vi "SPD Stand Operator UI.vi"() -> ()   [LabVIEW 2018]
uses:
  Instruments/KC705 DevBoard/typedefs/DevB.Message type.ctl
  Instruments/KeySight 53230A/typedefs/FreqC.Message Type.ctl
  Instruments/KC705 DevBoard/Message API/Send Message/DevB.Send Message I32.vi
  Instruments/KC705 DevBoard/Message API/Get Data/Variant to I32.vi
  Instruments/KC705 DevBoard/Message API/Get Data/Variant to Bool.vi
  Instruments/SPD HID Interface/hidSPDLibForLabView/hidSPDLibForLabView.lvlib
panel:
  out "FCount.Connected":bool caption="Connected"
  out "SPD.HeatsinkTempChart":sgl(graph)=40.51374 caption="Heatsink Temprature"
  out "SPD.DiodTempChart":sgl(graph)=-42.149345 caption="Diod Temprature"
  out "FCount.Count":dbl caption="Count" format="%#_12p"
  in  "FCount.Timed Totalize":dbl caption="Totalize time" format="%#_g Sec"
  in  "FCount.Level":dbl caption="Threshold" format="%#_g V"
  out "DevB.Connected":bool caption="Connected"
  in  "DevB.Delay":i32 caption="Delay"
  in  "DevB.Phase":i32 caption="Phase"
  in  "DevB.Frequency":i32 caption="Frequency"
  in  "DevB.Pulse Duration":i32 caption="Duration"
  out "error out":errorcluster
  out "UI Stoped":bool
  in  "Stop":bool
  # "KC705 DevBoard"
  # "Counter"
  # "Photon Detector"
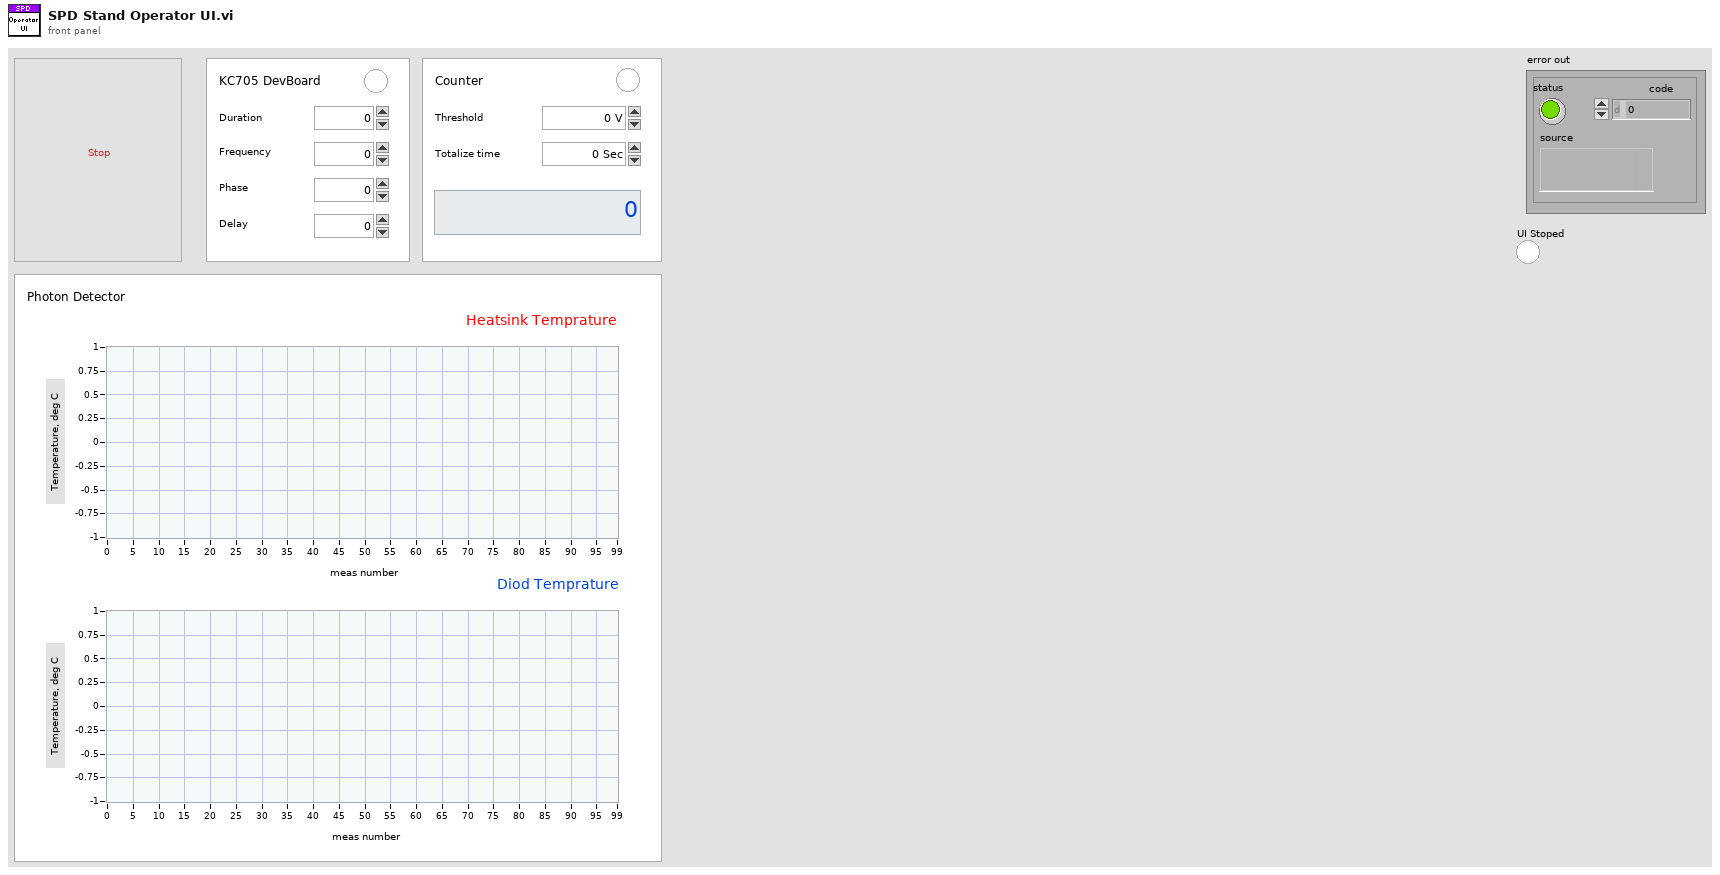
[diagram p1: front panel]
types:
  T1 = typedef "DevB.Message Session.ctl" = cluster{"Message queue":refnum<queue>, "stop event":refnum<user-event>}
  T2 = typedef "FreqC.Message Session.ctl" = cluster{"Message queue":refnum<queue>, "stop event":refnum<user-event>}
  T3 = typedef "hidSPDLibForLabView.lvlib/hidSPD HidDevInfo.ctl" = cluster{"name":string, "path":string}
  T4 = typedef "DevB.Session.ctl" = cluster{"DevBRef":refnum<visa-resource-name>, "connected":bool}
  T5 = typedef "hidSPDLibForLabView.lvlib/hidSPD Device Session.ctl" = cluster{"spdRef":u64, "connected":bool}
  T6 = typedef "FreqC.Session.ctl" = cluster{"FreqCRef":refnum<visa-resource-name>, "timeout":dbl, "connected":bool}
  T7 = typedef "DevB.Message type.ctl" = enum16{"Idle", "Set Duration", "Set Frequency", "Set Phase", "Set Delay", "on/off", "check status"}
  T8 = typedef "FreqC.Message Type.ctl" = enum16{"meas", "set level", "set gate"}
  T9 = typedef "hidSPDLibForLabView.lvlib/hidSPD Simple Report.ctl" = cluster{"Heatsink Temprature":sgl, "Diod Temprature":sgl, "TEC-voltage":sgl, "Diod Bias":sgl, "RF Power":sgl, "Thermal used":sgl, "hv bias used":sgl, "hv code used":u16, "strobe code used":u16, "SPD number":u8, "SPD ready":u8}
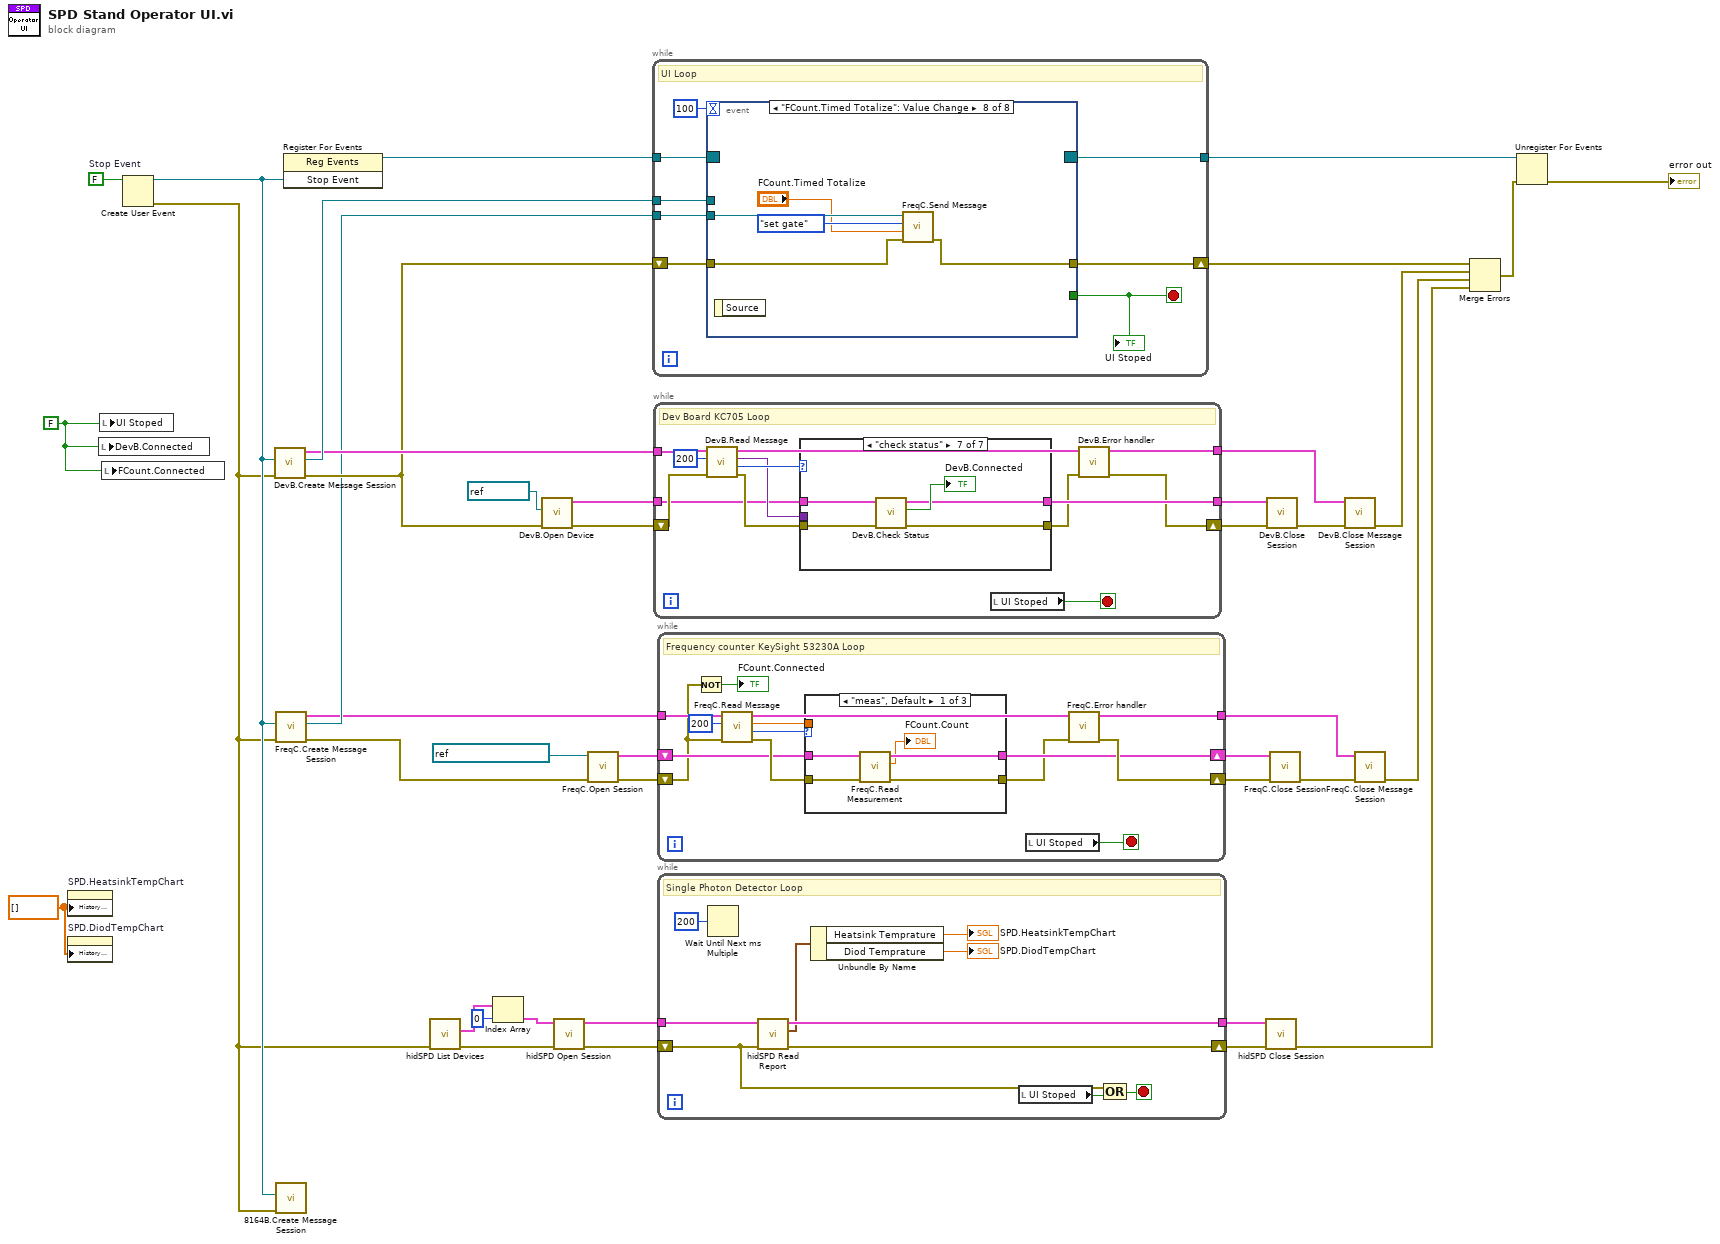
[diagram p0: block diagram]
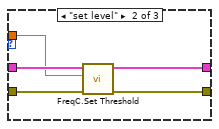
[diagram p2: hidden frame]
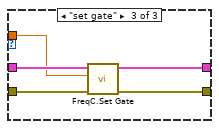
[diagram p3: hidden frame]
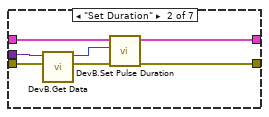
[diagram p5: hidden frame]
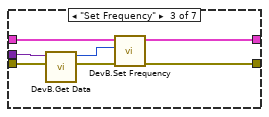
[diagram p6: hidden frame]
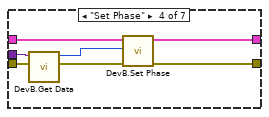
[diagram p7: hidden frame]
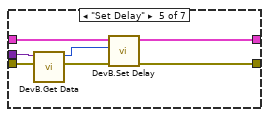
[diagram p8: hidden frame]
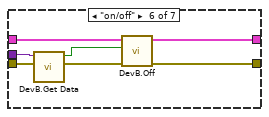
[diagram p9: hidden frame]
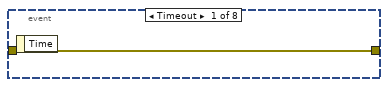
[diagram p10: hidden frame]
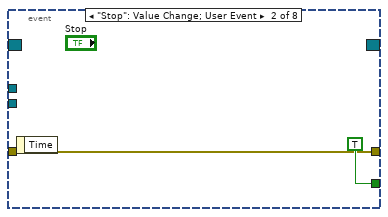
[diagram p11: hidden frame]
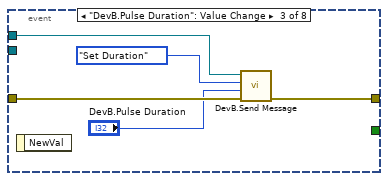
[diagram p12: hidden frame]
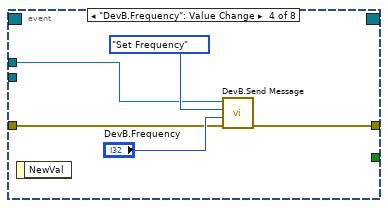
[diagram p13: hidden frame]
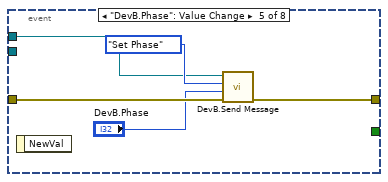
[diagram p14: hidden frame]
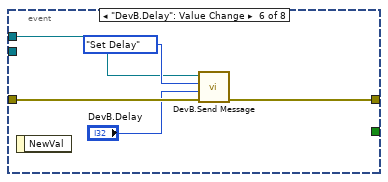
[diagram p15: hidden frame]
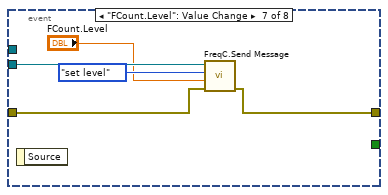
[diagram p16: hidden frame]
diagram:
  w4 = sgl[] [] ("History Data")
  w3 = FALSE ("UI Stoped")
  w41 = FALSE  # Stop Event
  n1 = property on="SPD.HeatsinkTempChart" class="WFChart (strict)"("History Data"=w4) -> ()  [unwired: 2 in, 2 out]
  n2 = property on="SPD.DiodTempChart" class="WFChart (strict)"("History Data"=w4) -> ()  [unwired: 2 in, 2 out]
  n3 = local write "DevB.Connected"(w3) -> ()
  n4 = local write "UI Stoped"(w3) -> ()
  n5 = local write "FCount.Connected"(w3) -> ()
  n6 = Create User Event(user event datatype=w41) -> (user event=w2:refnum<user-event>, error out=w1:errorcluster)  [unwired: 1 in]
  n7 = call "DevB.Create Message Session.vi"("error in"=w1, "stop event"=w2) -> ("error out"=w28:errorcluster, "DevB Message queue"=w39:refnum<queue>, "DevB Session out"=w31:T1)  [unwired: 7 in]
  n8 = call "FreqC.Create Message Session.vi"("error in"=w1, "stop event"=w2) -> ("error out"=w19:errorcluster, "FreqC Message queue"=w24:refnum<queue>, "FreqC Message Session out"=w21:T2)  [unwired: 7 in]
  n9 = call "8164B.Create Message Session.vi"("error in"=w1, "stop event"=w2) -> ()  [unwired: 7 in, 3 out]
  n10 = register-events(w2) -> (reference out=w40:refnum<event-registration>)  [unwired: 2 in, 1 out]
  n11 = call "hidSPD List Devices.vi"("error in (no error)"=w1) -> ("error out"=w10:errorcluster, "devices list"=w13:T3[])  [unwired: 9 in]
  n12 = Index Array(array=w13, index=0 ("index (row)")) -> (element=w12:T3)
  n13 = call "DevB.Open Device.vi"("error in (no error)"=w28, "Port"=refnum<visa-resource-name> "COM3") -> ("error out"=w35:errorcluster, "DevB Session out"=w36:T4)  [unwired: 8 in]
  n14 = call "hidSPD Open Session.vi"("error in (no error)"=w10, "HidDevInfo"=w12) -> ("error out"=w9:errorcluster, "spdDevSession out"=w8:T5)  [unwired: 8 in]
  n15 = call "FreqC.Open Session.vi"("error In"=w19, "VISA resource name"=refnum<visa-resource-name> "KeySight_53230A") -> ("error out"=w18:errorcluster, "FreqC Session out"=w17:T6)  [unwired: 8 in]
  n16 = while {
    tunnel: w40 -> [w47]
    tunnel: w39 -> [w45]
    tunnel: [w46] -> w33
    shift-right: [w43] -> w27
    shift-left: w28 -> [w44]
    tunnel: w24 -> [w42]
    stop <- w48 stop-if-true
    # "UI Loop"
    n17 = event shown="[7] \"FCount.Timed Totalize\": Value Change" {
      selector: w47 -> [_ _ _ _ _ _ _ _]
      dyn-events: [_ _ _ _ _ _ _ _] -> w46
      timeout: 100 -> [_ _ _ _ _ _ _ _]
      tunnel: [_ TRUE ("Stop") _ _ _ _ _ _] -> w48
      tunnel: w45 -> [_ _ w57 w61 w66 w71 _ _]
      tunnel: w44 -> [w50 w51 w55 w59 w65 w70 w74 w80]
      tunnel: [w50 w51 w53 w58 w63 w69 w73 w79] -> w43
      tunnel: w42 -> [_ _ _ _ _ _ w77 w82]
      event Timeout {
        n18 = event-data() -> ()  [unwired: 1 in, 1 out]
      }
      event "Stop": Value Change; User Event {
        n19 = event-data() -> ()  [unwired: 1 in, 1 out]
      }
      event "DevB.Pulse Duration": Value Change {
        n20 = event-data() -> ()  [unwired: 1 in, 1 out]
        n21 = call-poly "DevB.Send Message.vi"("error in (no error)"=w55, "data"="DevB.Pulse Duration", "Message"=DevB.Message_type."Set Duration", "DevB.Message queue in"=w57) -> ("error out"=w53:errorcluster)  [unwired: 6 in, 1 out]
      }
      event "DevB.Frequency": Value Change {
        n22 = event-data() -> ()  [unwired: 1 in, 1 out]
        n23 = call-poly "DevB.Send Message.vi"("error in (no error)"=w59, "data"="DevB.Frequency", "Message"=DevB.Message_type."Set Frequency", "DevB.Message queue in"=w61) -> ("error out"=w58:errorcluster)  [unwired: 6 in, 1 out]
      }
      event "DevB.Phase": Value Change {
        n24 = event-data() -> ()  [unwired: 1 in, 1 out]
        n25 = call-poly "DevB.Send Message.vi"("error in (no error)"=w65, "data"="DevB.Phase", "Message"=DevB.Message_type."Set Phase", "DevB.Message queue in"=w66) -> ("error out"=w63:errorcluster)  [unwired: 6 in, 1 out]
      }
      event "DevB.Delay": Value Change {
        n26 = event-data() -> ()  [unwired: 1 in, 1 out]
        n27 = call-poly "DevB.Send Message.vi"("error in (no error)"=w70, "data"="DevB.Delay", "Message"=DevB.Message_type."Set Delay", "DevB.Message queue in"=w71) -> ("error out"=w69:errorcluster)  [unwired: 6 in, 1 out]
      }
      event "FCount.Level": Value Change {
        n28 = event-data() -> ()  [unwired: 1 in, 1 out]
        n29 = call "FreqC.Send Message.vi"("error in"=w74, "data"="FCount.Level", "Message type"=FreqC.Message_Type."set level", "FreqC Message queue in"=w77) -> ("error out"=w73:errorcluster)  [unwired: 6 in, 1 out]
      }
      event "FCount.Timed Totalize": Value Change {
        n30 = event-data() -> ()  [unwired: 1 in, 1 out]
        n31 = call "FreqC.Send Message.vi"("error in"=w80, "data"="FCount.Timed Totalize", "Message type"=FreqC.Message_Type."set gate", "FreqC Message queue in"=w82) -> ("error out"=w79:errorcluster)  [unwired: 6 in, 1 out]
      }
    }
    "UI Stoped" <- w48
  }
  n32 = while {
    tunnel: [w91] -> w38
    tunnel: w36 -> [w87]
    tunnel: w31 -> [w88]
    tunnel: [w85] -> w29
    shift-right: [w83] -> w37
    shift-left: w35 -> [w94]
    stop <- w95 stop-if-true
    # "Dev Board KC705 Loop"
    n33 = call "DevB.Read Message.vi"("error in (no error)"=w94, "timeout in ms (-1)"=200, "DevB Session in"=w88) -> ("error out"=w90:errorcluster, "type"=w92:T7, "data"=w89:variant, "DevB Session out"=w86:T1)  [unwired: 5 in]
    n34 = case shown="\"check status\"" w92 {
      tunnel: w87 -> [w97 w99 w107 w113 w123 w130 w136]
      tunnel: [w97 w104 w106 w115 w120 w126 w134] -> w91
      tunnel: [w96 w103 w105 w114 w119 w127 w133] -> w84
      tunnel: w90 -> [w96 w102 w111 w117 w125 w132 w137]
      tunnel: w89 -> [_ w101 w110 w118 w124 w131 _]
      frame "Idle", Default {
      }
      frame "Set Duration" {
        n35 = call-poly "DevB.Get Data.vi"("error in"=w102, "data variant"=w101) -> ("error out"=w98:errorcluster, "data out"=w100:i32)  [unwired: 8 in]
        n36 = call "DevB.Set Pulse Duration.vi"("error in (no error)"=w98, "Pulse Duration"=w100, "DevB Session in"=w99) -> ("error out"=w103:errorcluster, "DevB Session out"=w104:T4)  [unwired: 7 in]
      }
      frame "Set Frequency" {
        n37 = call-poly "DevB.Get Data.vi"("error in"=w111, "data variant"=w110) -> ("error out"=w109:errorcluster, "data out"=w108:i32)  [unwired: 8 in]
        n38 = call "DevB.Set Frequency.vi"("error in (no error)"=w109, "Frequency"=w108, "DevB Session in"=w107) -> ("error out"=w105:errorcluster, "DevB Session out"=w106:T4)  [unwired: 7 in]
      }
      frame "Set Phase" {
        n39 = call-poly "DevB.Get Data.vi"("error in"=w117, "data variant"=w118) -> ("error out"=w112:errorcluster, "data out"=w116:i32)  [unwired: 8 in]
        n40 = call "DevB.Set Phase.vi"("error in (no error)"=w112, "Phase"=w116, "DevB Session in"=w113) -> ("error out"=w114:errorcluster, "DevB Session out"=w115:T4)  [unwired: 7 in]
      }
      frame "Set Delay" {
        n41 = call-poly "DevB.Get Data.vi"("error in"=w125, "data variant"=w124) -> ("error out"=w122:errorcluster, "data out"=w121:i32)  [unwired: 8 in]
        n42 = call "DevB.Set Delay.vi"("error in (no error)"=w122, "Delay"=w121, "DevB Session in"=w123) -> ("error out"=w119:errorcluster, "DevB Session out"=w120:T4)  [unwired: 7 in]
      }
      frame "on/off" {
        n43 = call-poly "DevB.Get Data.vi"("error in"=w132, "data variant"=w131) -> ("error out"=w129:errorcluster, "data out"=w128:bool)  [unwired: 8 in]
        n44 = call "DevB.Off.vi"("error in (no error)"=w129, "off"=w128, "DevB Session in"=w130) -> ("error out"=w127:errorcluster, "DevB Session out"=w126:T4)  [unwired: 7 in]
      }
      frame "check status" {
        n45 = call "DevB.Check Status.vi"("error in (no error)"=w137, "DevB Session in"=w136) -> ("error out"=w133:errorcluster, "Connected"=→"DevB.Connected":bool, "DevB Session out"=w134:T4)  [unwired: 7 in]
      }
    }
    n46 = local read "UI Stoped"() -> (w95:bool)
    n47 = call "DevB.Error handler.vi"("error in (no error)"=w84, "DevB Session in"=w86) -> ("error out"=w83:errorcluster, "DevB Session out"=w85:T1)  [unwired: 8 in]
  }
  n48 = while {
    tunnel: w21 -> [w148]
    shift-right: [w149] -> w15
    shift-left: w18 -> [w138]
    tunnel: [w150] -> w22
    shift-right: [w142] -> w16
    shift-left: w17 -> [w143]
    stop <- w151 stop-if-true
    # "Frequency counter KeySight 53230A Loop"
    n49 = Not(x=w138) -> (.not. x?=→"FCount.Connected":bool)
    n50 = call "FreqC.Read Message.vi"("error in (no error)"=w138, "timeout in ms (-1)"=200, "FreqC Message Session in"=w148) -> ("error out"=w144:errorcluster, "type"=w146:T8, "data"=w141:dbl, "FreqC Message Session out"=w147:T2)  [unwired: 5 in]
    n51 = case shown="\"meas\", Default" w146 {
      tunnel: w144 -> [w155 w159 w164]
      tunnel: w143 -> [w156 w161 w166]
      tunnel: [w154 w157 w163] -> w140
      tunnel: [w153 w158 w162] -> w142
      tunnel: w141 -> [_ w160 w165]
      frame "meas", Default {
        n52 = call "FreqC.Read Measurement.vi"("error In"=w155, "FreqC Session in"=w156) -> ("error out"=w154:errorcluster, "Measurement"=→"FCount.Count":dbl, "FreqC Session out"=w153:T6)  [unwired: 7 in]
      }
      frame "set level" {
        n53 = call "FreqC.Set Threshold.vi"("error In"=w159, "Threshold, V"=w160, "FreqC Session in"=w161) -> ("error out"=w157:errorcluster, "FreqC Session out"=w158:T6)  [unwired: 7 in]
      }
      frame "set gate" {
        n54 = call "FreqC.Set Gate.vi"("error In"=w164, "Gate, sec"=w165, "FreqC Session in"=w166) -> ("error out"=w163:errorcluster, "FreqC Session out"=w162:T6)  [unwired: 7 in]
      }
    }
    n55 = local read "UI Stoped"() -> (w151:bool)
    n56 = call "FreqC.Error handler.vi"("error in"=w140, "FreqC Message Session in"=w147) -> ("error out"=w149:errorcluster, "FreqC Message Session out"=w150:T2)  [unwired: 8 in]
  }
  n57 = while {
    tunnel: w8 -> [w175]
    tunnel: [w174] -> w7
    shift-right: [w172] -> w5
    shift-left: w9 -> [w167]
    stop <- w168 stop-if-true
    # "Single Photon Detector Loop"
    n58 = Wait Until Next ms Multiple(millisecond multiple=u32 200) -> ()  [unwired: 1 out]
    n59 = call "hidSPD Read Report.vi"("error in (no error)"=w167, "spdDevSession in"=w175) -> ("error out"=w172:errorcluster, "hidSPD Simple Report"=w171:T9, "spdDevSession out"=w174:T5)  [unwired: 7 in]
    n60 = Unbundle By Name(w171) -> ("Heatsink Temprature"=→"SPD.HeatsinkTempChart":sgl, "Diod Temprature"=→"SPD.DiodTempChart":sgl)
    n61 = local read "UI Stoped"() -> (w176:bool)
    n62 = Compound Arithmetic op=OR(w167, w176) -> (w168:bool)
  }
  n63 = call "hidSPD Close Session.vi"("error in (no error)"=w5, "spdDevHandle"=w7) -> ("error out"=w6:errorcluster)  [unwired: 9 in]
  n64 = call "DevB.Close Session.vi"("error in (no error)"=w37, "DevB Session"=w38) -> ("error out"=w30:errorcluster)  [unwired: 9 in]
  n65 = call "FreqC.Close Session.vi"("error In"=w15, "FreqC Session in"=w16) -> ("error out"=w14:errorcluster)  [unwired: 9 in]
  n66 = call "DevB.Close Message Session.vi"("error in"=w30, "DevBoard Message session"=w29) -> ("error out"=w26:errorcluster)  [unwired: 9 in]
  n67 = call "FreqC.Close Message Session.vi"("error in"=w14, "FreqC Message Session in"=w22) -> ("error out"=w23:errorcluster)  [unwired: 9 in]
  n68 = Merge Errors(w27, w26, w23, w6) -> (w25:errorcluster)
  n69 = Unregister For Events(event registration refnum=w33, error in=w25) -> (error out=→"error out":errorcluster)
